vi "InitDataEvent.vi"(8 "error in (no error)":errorcluster, 9 "data":T12, 10 "Ir Data Event":T9, 11 "config":T15) -> (0 "error out":errorcluster, 2 "data event":T1)   [LabVIEW 2017, in "IrDataEventCreator.lvlib"]
uses:
  <vilib>/addons/InsightCM/Devices/Shared/Ir/IrDataEventCreator/IrDataEventCreator.lvlib
  <vilib>/addons/InsightCM/Devices/Shared/Ir/IrDataEventCreator/controls/config.ctl
  <vilib>/addons/InsightCM/Devices/Shared/Common/DataFlow/controls/Data.ctl
  <vilib>/addons/InsightCM/Utilities/DataAccessors/controls/wfmSGL_DVR.ctl
  <vilib>/addons/PointValueMap/controls/PointMap.ctl
  <vilib>/addons/InsightCM/Devices/Shared/Common/DataFlow/controls/Type.ctl
  <vilib>/addons/InsightCM/Devices/Shared/Ir/IrDataEventCreator/controls/IrDataEvent.ctl
  <vilib>/addons/InsightCM/Devices/Shared/Common/DataEvent/controls/EventReference.ctl
  <vilib>/addons/InsightCM/Devices/Shared/Common/DataEvent/controls/Event.ctl
  <vilib>/addons/InsightCM/MessageBus/Base/controls/DataEvent.ctl
  <vilib>/addons/InsightCM/MessageBus/Base/controls/KeyValuePair.ctl
  <vilib>/addons/InsightCM/Devices/Shared/Common/DataEvent/controls/DataSet.ctl
  <vilib>/addons/InsightCM/MessageBus/Base/controls/DataSetMetadata.ctl
  <vilib>/addons/InsightCM/MessageBus/Base/controls/TrendPoint.ctl
  <vilib>/addons/InsightCM/MessageBus/Base/controls/TrendAlarmUpdate.ctl
  <vilib>/addons/InsightCM/MessageBus/Base/controls/TrendAlarmTransition.ctl
  <vilib>/addons/InsightCM/SRP/SRP.lvlib
  <vilib>/addons/InsightCM/Devices/Shared/Common/DataEvent/DataEvent.lvlib
  <vilib>/addons/PointValueMap/PointValueMap.lvlib
  <vilib>/addons/InsightCM/Devices/Shared/Common/DataFlow/DataFlow.lvlib
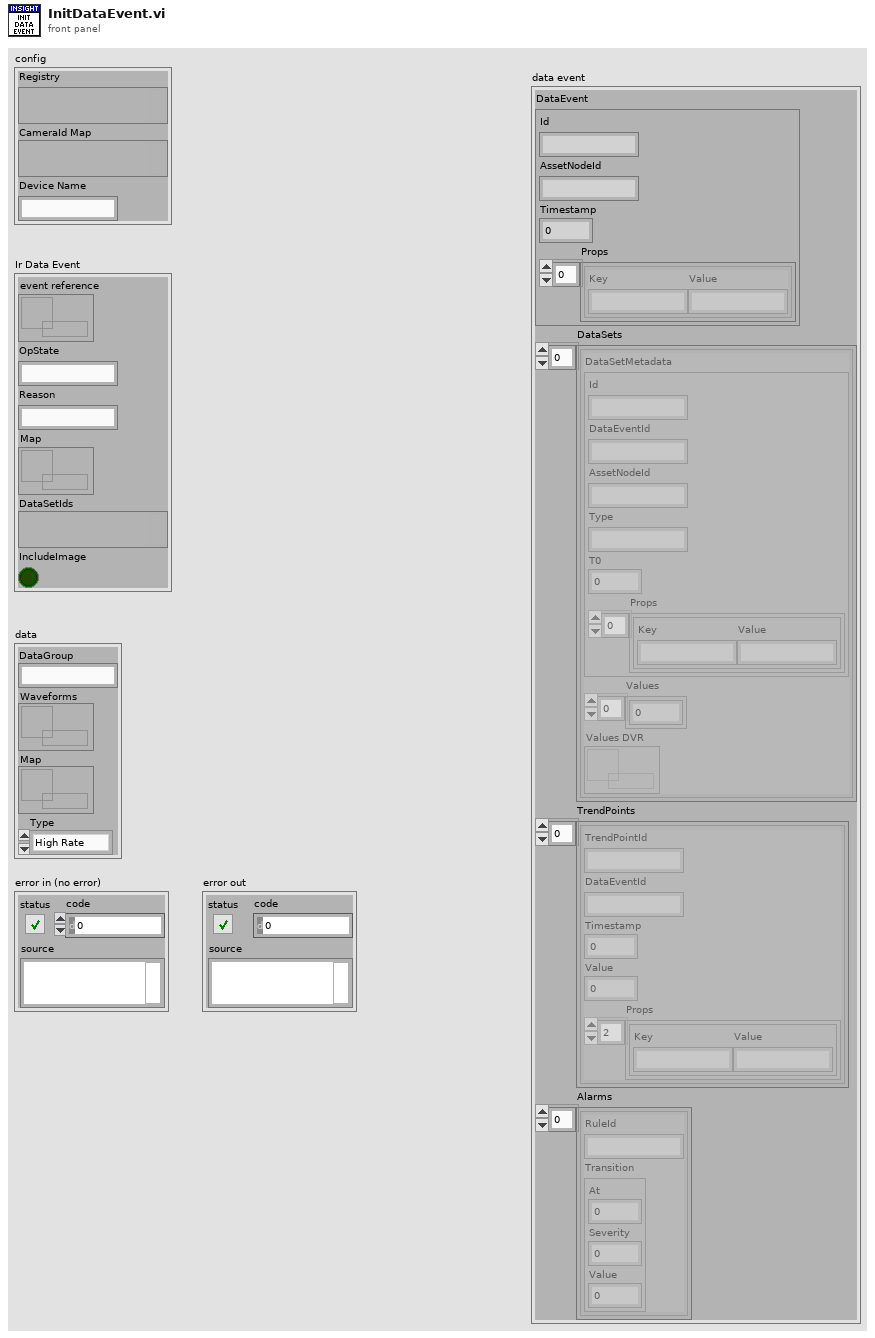
[diagram p1: front panel]
types:
  T1 = typedef "DataEvent.lvlib/Event.ctl" = cluster{"DataEvent":T2, "DataSets":T4[], "TrendPoints":T6[], "Alarms":T7[]}
  T2 = typedef "DataEvent.ctl" = cluster{"Id":string, "AssetNodeId":string, "Timestamp":i64, "Props":T3[]}
  T3 = typedef "KeyValuePair.ctl" = cluster{"Key":string, "Value":string}
  T4 = typedef "DataEvent.lvlib/DataSet.ctl" = cluster{"DataSetMetadata":T5, "Values":sgl[], "Values DVR":refnum<data-value>}
  T5 = typedef "DataSetMetadata.ctl" = cluster{"Id":string, "DataEventId":string, "AssetNodeId":string, "Type":string, "T0":i64, "Props":T3[]}
  T6 = typedef "TrendPoint.ctl" = cluster{"TrendPointId":string, "DataEventId":string, "Timestamp":i64, "Value":dbl, "Props":T3[]}
  T7 = typedef "TrendAlarmUpdate.ctl" = cluster{"RuleId":string, "Transition":T8}
  T8 = typedef "TrendAlarmTransition.ctl" = cluster{"At":i64, "Severity":i32, "Value":dbl}
  T9 = typedef "IrDataEventCreator.lvlib/IrDataEvent.ctl" = cluster{"event reference":T10, "OpState":string, "Reason":string, "Map":T11, "DataSetIds":variant, "IncludeImage":bool}
  T10 = typedef "DataEvent.lvlib/EventReference.ctl" = refnum<data-value>
  T11 = typedef "PointValueMap.lvlib/PointMap.ctl" = refnum<data-value>
  T12 = typedef "DataFlow.lvlib/Data.ctl" = cluster{"DataGroup":string, "Waveforms":T13, "Map":T11, "Type":T14}
  T13 = typedef "wfmSGL_DVR.ctl" = refnum<data-value>
  T14 = typedef "DataFlow.lvlib/Type.ctl" = enum16{"High Rate", "Low Rate", "Burst Mode"}
  T15 = typedef "IrDataEventCreator.lvlib/config.ctl" = cluster{"Registry":variant, "CameraId Map":variant, "Device Name":string}
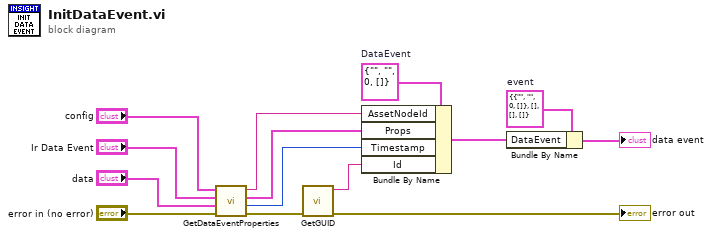
[diagram p0: block diagram]
diagram:
  w13 = T2 {"Id"="", "AssetNodeId"="", "Timestamp"=0, "Props"=[]}  # DataEvent
  w14 = T1 {"DataEvent"={"Id"="", "AssetNodeId"="", "Timestamp"=0, "Props"=[]}, "DataSets"=[], "TrendPoints"=[], "Alarms"=[]}  # event
  n1 = call <vilib>:"GetDataEventProperties.vi"("error in (no error)"="error in (no error)", "data"="data", "Ir Data Event"="Ir Data Event", "config"="config") -> ("error out"=w7:errorcluster, "Timestamp"=w11:i64, "Props"=w10:T3[], "AssetNodeId"=w4:string)  [unwired: 4 in]
  n2 = call <vilib>:"GetGUID.vi"("error in (no error)"=w7) -> ("error out"=→"error out":errorcluster, "GUID"=w12:string)  [unwired: 9 in]
  n3 = Bundle By Name(cluster=w13, "AssetNodeId"=w4, "Props"=w10, "Timestamp"=w11, "Id"=w12) -> (w2:T2)
  n4 = Bundle By Name(cluster=w14, "DataEvent"=w2) -> (→"data event":T1)
